vi "Wire Init Terms.vi"(6 "State":T1={"Worker Library Path"=path "", "Block Label"="", "Types"=[], "Selections"=[], "Icon"={"image type"=0, "image depth"=0, "image"=[], "mask"=[], "colors"=[], "Rectangle"={"left"=0, "top"=0, "right"=0, "bottom"=0}}, "Errors"={"Terminals"=[], "Generate"={"status"=FALSE, "code"=0, "source"=""}, "General"={"status"=FALSE, "code"=0, "source"=""}}, "Calculated Sizes"={"Block Width"=0, "Block Height"=0, "Half Width"=0, "Icon Top"=0, "Icon Bottom"=0, "Label Width"=0, "Half Label"=0, "Label Top"=0, "Text Width"=0, "Half Text"=0, "Text Height"=0, "Label Height"=0, "Expanded Width"=0, "Label Bottom"=0, "Expanded Top"=0, "Expanded Bottom"=0, "Expanded Height"=0, "Min Height"=0, "Max Height"=0}, "Special Terminal Indices"={"Action"=-1, "Init"=-1, "Tag"=-1, "State in"=-1, "State out"=-1, "Error"=-1}, "Terminals"=[]}, 8 "error in (no error)":errorcluster, 10 "Grouped Terms":T13, 11 "Refs In":T15) -> (0 "error out":errorcluster, 3 "Refs":T15)   [LabVIEW 2022 SP3, in "FlexBlocks Support.lvlib"]
uses:
  FlexBlocks Support.lvlib
  SM Refs.ctl
  Grouped Terms.ctl
  Terminal Group.ctl
  Type Descriptor.ctl
  Terminal Direction.ctl
  Value Mode.ctl
  Special Terminal.ctl
  Terminal State.ctl
  Flex Block/State.ctl
  <vilib>/picture/picture.llb/imagedata.ctl
  XNode Errors.ctl
  Calculated Sizes.ctl
  Special Terminal Indices.ctl
  Terminal Status.ctl
  Terminal Draw Style.ctl
  Flex Block/Flex Block.xnode
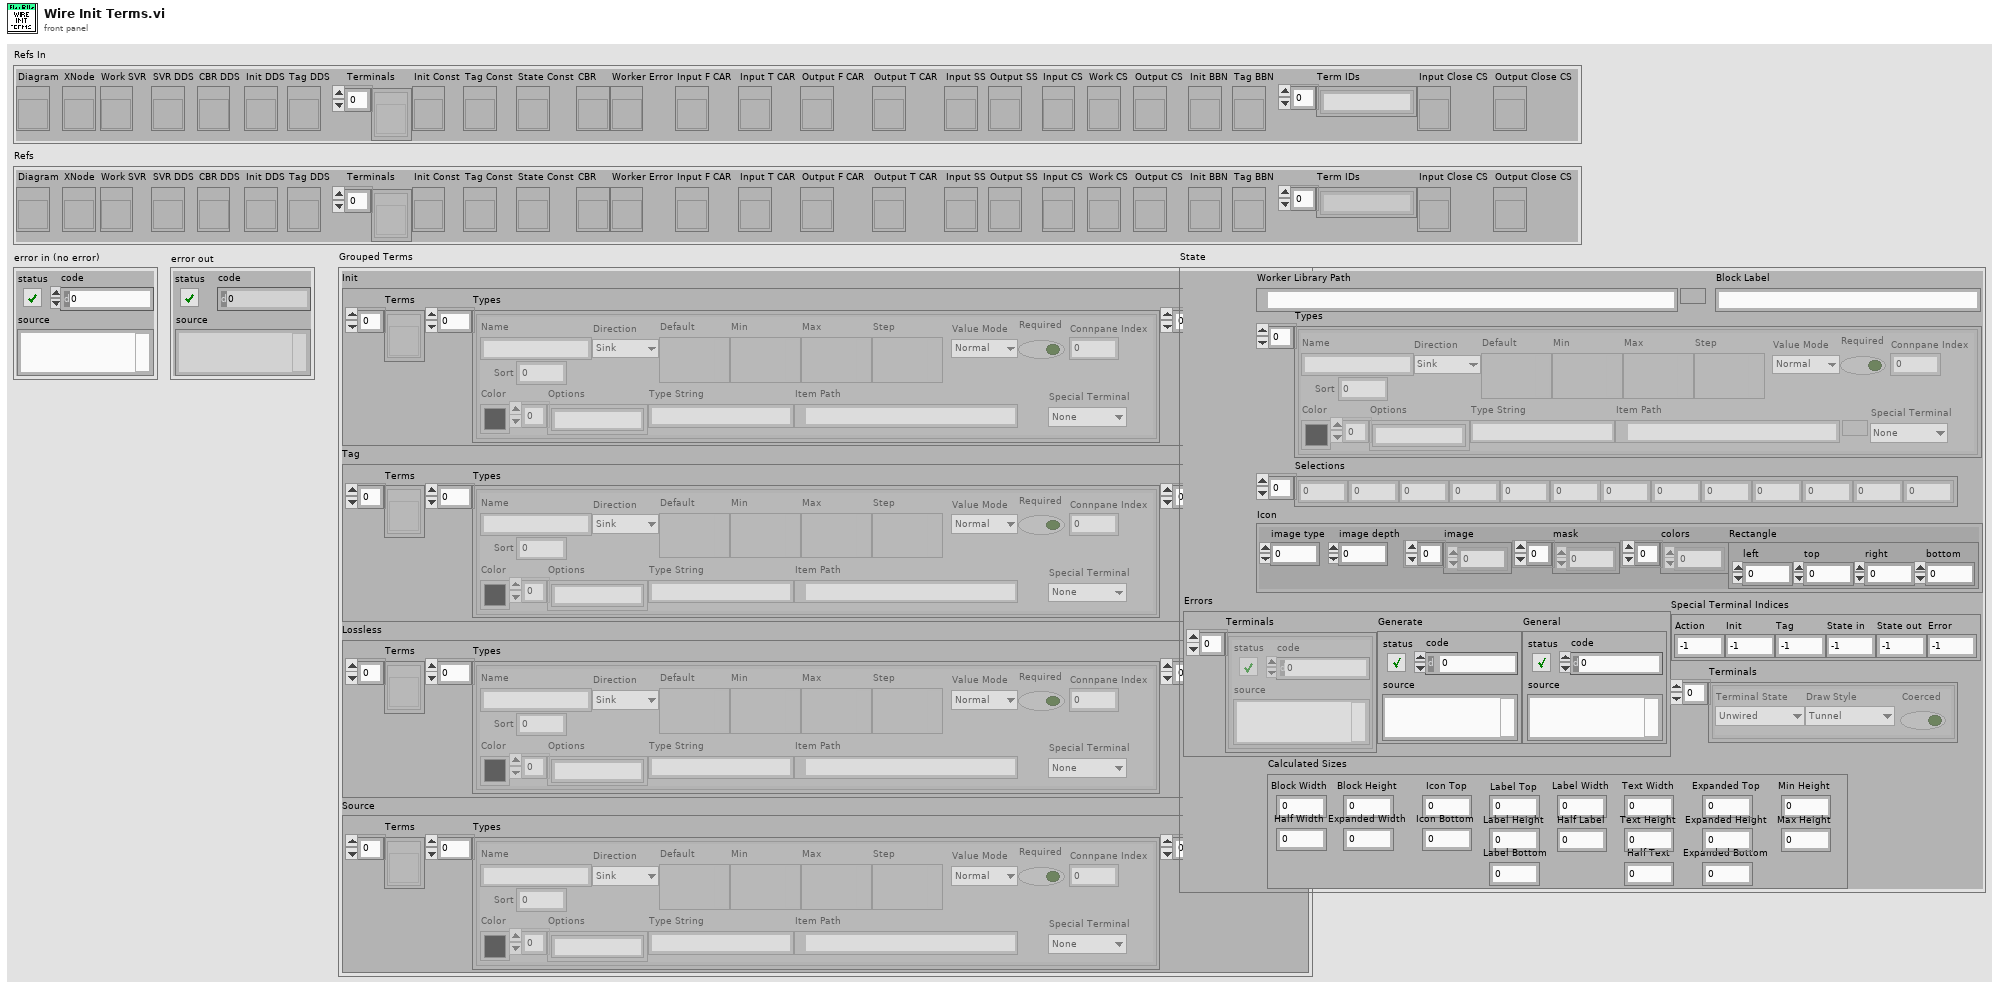
[diagram p1: front panel]
types:
  T1 = typedef "Flex Block.xnode/State.ctl" = cluster{"Worker Library Path":path, "Block Label":string, "Types":T2[], "Selections":i32[], "Icon":T6, "Errors":T7, "Calculated Sizes":T8, "Special Terminal Indices":T9, "Terminals":T10[]}
  T2 = typedef "FlexBlocks Support.lvlib/Type Descriptor.ctl" = cluster{"Name":string, "Direction":T3, "Default":variant, "Min":variant, "Max":variant, "Step":variant, "Value Mode":T4, "Color":u32, "Options":string[], "Type String":string, "Item Path":path, "Required":bool, "Connpane Index":i32, "Special Terminal":T5, "Sort":i32}
  T3 = typedef "FlexBlocks Support.lvlib/Terminal Direction.ctl" = enum16{"Sink", "Source"}
  T4 = typedef "FlexBlocks Support.lvlib/Value Mode.ctl" = enum16{"Normal", "Range", "Select"}
  T5 = typedef "FlexBlocks Support.lvlib/Special Terminal.ctl" = enum16{"None", "Action", "Init", "Tag", "State in", "State out", "Error"}
  T6 = typedef "imagedata.ctl" = cluster{"image type":i32, "image depth":i32, "image":u8[], "mask":u8[], "colors":u32[], "Rectangle":cluster{"left":i16, "top":i16, "right":i16, "bottom":i16}}
  T7 = typedef "FlexBlocks Support.lvlib/XNode Errors.ctl" = cluster{"Terminals":errorcluster[], "Generate":errorcluster, "General":errorcluster}
  T8 = typedef "FlexBlocks Support.lvlib/Calculated Sizes.ctl" = cluster{"Block Width":i32, "Block Height":i32, "Half Width":i32, "Icon Top":i32, "Icon Bottom":i32, "Label Width":i32, "Half Label":i32, "Label Top":i32, "Text Width":i32, "Half Text":i32, "Text Height":i32, "Label Height":i32, "Expanded Width":i32, "Label Bottom":i32, "Expanded Top":i32, "Expanded Bottom":i32, "Expanded Height":i32, "Min Height":i32, "Max Height":i32}
  T9 = typedef "FlexBlocks Support.lvlib/Special Terminal Indices.ctl" = cluster{"Action":i32, "Init":i32, "Tag":i32, "State in":i32, "State out":i32, "Error":i32}
  T10 = typedef "FlexBlocks Support.lvlib/Terminal Status.ctl" = cluster{"Terminal State":T11, "Draw Style":T12, "Coerced":bool}
  T11 = typedef "FlexBlocks Support.lvlib/Terminal State.ctl" = enum16{"Unwired", "BadType", "BadRef", "Channel", "Value", "Control Ref"}
  T12 = typedef "FlexBlocks Support.lvlib/Terminal Draw Style.ctl" = enum16{"Tunnel", "BadType", "BadRef", "Channel", "Value", "Control Ref"}
  T13 = typedef "FlexBlocks Support.lvlib/Grouped Terms.ctl" = cluster{"Init":T14, "Tag":T14, "Lossless":T14, "Source":T14}
  T14 = typedef "FlexBlocks Support.lvlib/Terminal Group.ctl" = cluster{"Terms":refnum<vi>[], "Types":T2[], "Wire Type":T11[]}
  T15 = typedef "FlexBlocks Support.lvlib/SM Refs.ctl" = cluster{"Diagram":refnum<vi>, "XNode":refnum<vi>, "Work SVR":refnum<vi>, "SVR DDS":refnum<vi>, "CBR DDS":refnum<vi>, "Init DDS":refnum<vi>, "Tag DDS":refnum<vi>, "Terminals":refnum<vi>[], "Init Const":refnum<vi>, "Tag Const":refnum<vi>, "State Const":refnum<vi>, "CBR":refnum<vi>, "Worker Error":refnum<vi>, "Input F CAR":refnum<vi>, "Input T CAR":refnum<vi>, "Output F CAR":refnum<vi>, "Output T CAR":refnum<vi>, "Input SS":refnum<vi>, "Output SS":refnum<vi>, "Input CS":refnum<vi>, "Work CS":refnum<vi>, "Output CS":refnum<vi>, "Init BBN":refnum<vi>, "Tag BBN":refnum<vi>, "Term IDs":string[], "Input Close CS":refnum<vi>, "Output Close CS":refnum<vi>}
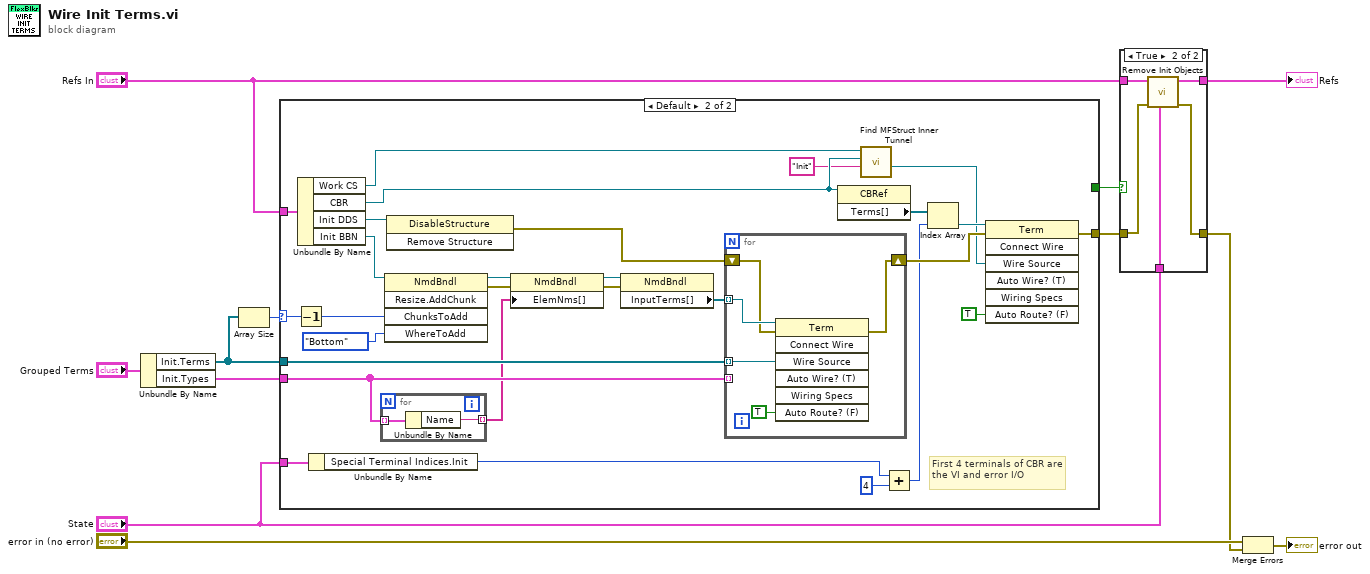
[diagram p0: block diagram]
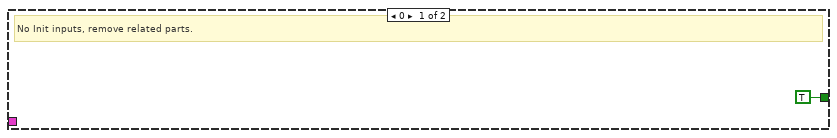
[diagram p3: hidden frame]
diagram:
  n1 = Unbundle By Name("Grouped Terms") -> ("Init.Terms"=w10:refnum<vi>[], "Init.Types"=w11:T2[])
  n2 = Array Size(array=w10) -> (size(s)=w9:i32)
  n3 = case shown="Default" w9 {
    selector: w9 -> [_ w35]
    tunnel: w11 -> [_ w29]
    tunnel: w10 -> [_ w39]
    tunnel: "Refs In" -> [_ w38]
    tunnel: "State" -> [_ w25]
    tunnel: [_ w15] -> w6
    tunnel: [TRUE _] -> w2
    frame 0 {
      # "No Init inputs, remove related parts."
    }
    frame Default {
      # "First 4 terminals of CBR are the VI and error I/O"
      n4 = Decrement(x=w35) -> (x-1=w34:i32)
      n5 = Unbundle By Name(w38) -> ("Work CS"=w21:refnum<vi>, "CBR"=w20:refnum<vi>, "Init DDS"=w37:refnum<vi>, "Init BBN"=w36:refnum<vi>)
      n6 = Unbundle By Name(w25) -> ("Special Terminal Indices.Init"=w23:i32)
      n7 = for {
        tunnel: w29 -> [w43] mode=indexing
        tunnel: [w42] -> w28 mode=indexing
        n8 = Unbundle By Name(w43) -> ("Name"=w42:string)
      }
      n9 = invoke class="NmdBndl" method="Resize.AddChunk"(reference=w36, "ChunksToAdd"=w34, "WhereToAdd"=enum8{"Bottom", "Top"}."Bottom" ("Where To Add")) -> (reference out=w31:refnum<vi>, error out=w30:errorcluster)  [unwired: 2 in, 3 out]
      n10 = invoke class="DisableStructure" method="Remove Structure"(reference=w37) -> (error out=w40:errorcluster)  [unwired: 2 in, 2 out]
      n11 = property class="NmdBndl"(reference=w31, error in=w30, "ElemNms[]"=w28) -> (reference out=w32:refnum<vi>, error out=w26:errorcluster)
      n12 = property class="NmdBndl"(reference=w32, error in=w26) -> ("InputTerms[]"=w27:refnum<vi>[])  [unwired: 2 out]
      n13 = for {
        tunnel: w39 -> [w47] mode=indexing
        tunnel: w29 -> [_] mode=indexing
        tunnel: w27 -> [w48] mode=indexing
        shift-right: [w45] -> w41
        shift-left: w40 -> [w46]
        n14 = invoke class="Term" method="Connect Wire"(reference=w48, error in=w46, "Wire Source"=w47, "Auto Route? (F)"=TRUE) -> (error out=w45:errorcluster)  [unwired: 3 in, 6 out]
      }
      n15 = property class="CBRef"(reference=w20) -> ("Terms[]"=w24:refnum<vi>[])  [unwired: 1 in, 2 out]
      n16 = call "Find MFStruct Inner Tunnel.vi"("Tunnel Name"="Init", "Contained GObject"=w20, "MFStruct"=w21) -> ("Inside Tunnel"=w16:refnum<vi>)  [unwired: 5 in, 3 out]
      n17 = Add(x=w23, y=4) -> (x+y=w18:i32)
      n18 = Index Array(array=w24, index=w18) -> (element=w17:refnum<vi>)
      n19 = invoke class="Term" method="Connect Wire"(reference=w17, error in=w41, "Wire Source"=w16, "Auto Route? (F)"=TRUE) -> (error out=w15:errorcluster)  [unwired: 3 in, 6 out]
    }
  }
  n20 = case shown="True" w2 {
    tunnel: w6 -> [w49 w54]
    tunnel: "Refs In" -> [w50 w55]
    tunnel: "State" -> [_ w53]
    tunnel: [w50 w52] -> w3
    tunnel: [w49 w51] -> w1
    frame False {
    }
    frame True {
      n21 = call "Remove Init Objects.vi"("State"=w53, "error in (no error)"=w54, "Refs In"=w55) -> ("error out"=w51:errorcluster, "Refs"=w52:T15)  [unwired: 7 in]
    }
  }
  "Refs" <- w3
  n22 = Merge Errors("error in (no error)", w1) -> (→"error out":errorcluster)
